vi "Read Keys.vi"(8 "error in (no error)":errorcluster, 11 "Section 2 in":refnum<class "Section 2.lvclass">) -> (0 "error out":errorcluster, 2 "Keys":cluster{"Name":string, "Value":string}[](array[cluster]), 3 "Section 2 out":refnum<class "Section 2.lvclass">)   [LabVIEW 2015, in "LVOOP Introduction.lvlib" / "Section 2.lvclass"]
doc: "Thi VI returns an array of key/values pairs of section.\n\nOverwriting dynamic dispatch VI."
uses:
  Section 2.lvclass
  Read String 1.vi
  Read String 2.vi
  Configuration/Classes/Section/Section.lvclass
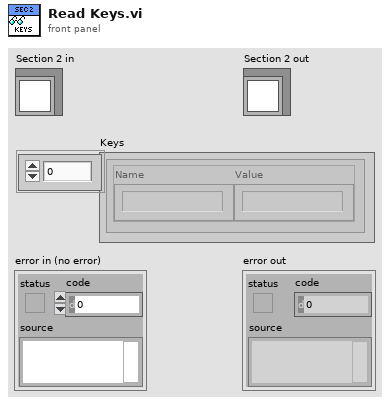
[diagram p1: front panel]
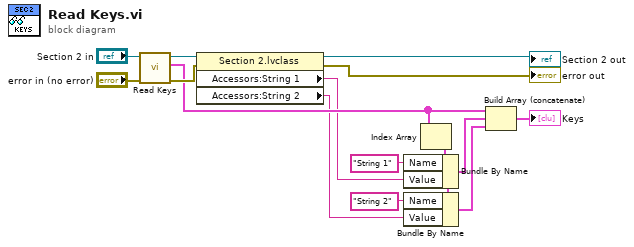
[diagram p0: block diagram]
diagram:
  n1 = call-parent "Read Keys.vi"("error in (no error)"="error in (no error)", "Section in"="Section 2 in") -> ("error out"=w7:errorcluster, "Keys"=w6:cluster{"Name":string, "Value":string}[], "Section out"=w10:refnum<class "Section 2.lvclass">)  [unwired: 7 in]
  n2 = property class="Section 2.lvclass"(reference=w10, error in=w7) -> (reference out=→"Section 2 out":refnum<class "Section 2.lvclass">, error out=→"error out":errorcluster, "Accessors:String 1"=w4:string, "Accessors:String 2"=w3:string)
  n3 = Index Array(array=w6) -> (element=w2:cluster{"Name":string, "Value":string})  [unwired: 1 in]
  n4 = Bundle By Name(cluster=w2, "Name"="String 1", "Value"=w4) -> (w11:cluster{"Name":string, "Value":string})
  n5 = Bundle By Name(cluster=w2, "Name"="String 2", "Value"=w3) -> (w1:cluster{"Name":string, "Value":string})
  n6 = Build Array (concatenate)(w6, w11, w1) -> (→"Keys":cluster{"Name":string, "Value":string}[])
